vi "test_Create Data Channel_array enumerated list.vi"(8 "error in (no error)":errorcluster, 11 "TestCase in":refnum<class "Instrument Addon Scripting API Channels Unit Tests.lvclass">) -> (0 "error out":errorcluster, 3 "TestCase out":refnum<class "Instrument Addon Scripting API Channels Unit Tests.lvclass">)   [LabVIEW 2020, in "Instrument Addon Scripting API Channels Unit Tests.lvclass"]
uses:
  Instrument Addon Scripting API Channels Unit Tests.lvclass
  APIs/Scripting API/TypeDefs/Array Enumerated List Settings.ctl
  APIs/Scripting API/TypeDefs/Array Element.ctl
  Addon/Addon Shared/Types/Protocol Data Type.ctl
  Addon/Addon Shared/Types/Data Channel Type.ctl
  Instrument Addon Scripting API Channels Unit Tests.lvclass/Instrument Addon Scripting API Channels Unit Tests.ctl
  Addon/Addon Shared/SubVIs/Constants.vi
  <vilib>/NI/NI VeriStand Advanced SysDef API/_SubVIs/SysDef.Search.GUID.vi
  <vilib>/NI/NI VeriStand Advanced SysDef API/_SubVIs/SysDef.Search.GUIDs.vi
  APIs/Scripting API/Channels/Create Data Channel - Array - Enumerated List.vi
  <vilib>/NI VeriStand/Custom Device API/Get Item Property (U16).vi
  <vilib>/addons/_JKI Toolkits/VI Tester/TestCase.llb/TestCase.lvclass
  <vilib>/NI/NI VeriStand Advanced SysDef API/SysDef API/Advanced System Definition.lvlib
  Addon/Addon Shared/Instrument Addon Shared.lvlib
  APIs/Scripting API/Instrument Addon Scripting API.lvlib
  <vilib>/NI VeriStand/Custom Device API/Custom Device API.lvlib
  C:/Program Files (x86)/National Instruments/LabVIEW 2020/vi.lib/addons/_JKI Toolkits/VI Tester/TestCase.llb/TestCase.lvclass
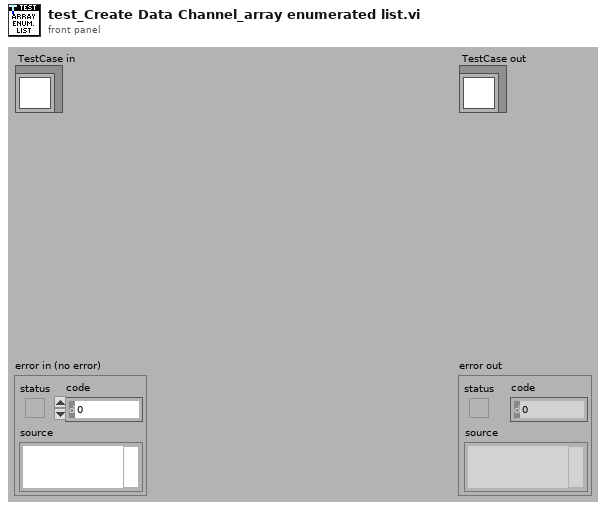
[diagram p1: front panel]
types:
  T1 = typedef "Instrument Addon Scripting API.lvlib/Array Enumerated List Settings.ctl" = cluster{"Elements":T2[], "Enumerated List":string[], "Delimiter":string}
  T2 = typedef "Instrument Addon Scripting API.lvlib/Array Element.ctl" = cluster{"Name":string, "Default Value":dbl, "Units":string}
  T3 = typedef "Instrument Addon Shared.lvlib/Data Channel Type.ctl" = enum16{"Format", "Comparison", "Type Cast", "Enumerated List"}
  T4 = typedef "Instrument Addon Shared.lvlib/Protocol Data Type.ctl" = enum16{"Single Channel", "Array"}
  T5 = typedef "Custom Device API.lvlib/Custom Device Item Ref.ctl" = u64
  T6 = typedef "Advanced System Definition.lvlib/TreeItem.Info.ctl" = cluster{"Name":string, "Description":string, "GUID":string, "Is Channel":bool, "Channel":T7, "Is Waveform":bool, "Waveform":T9}
  T7 = typedef "Custom Device API.lvlib/Custom Device Channel.ctl" = cluster{"Type":T8, "Units":string, "Default Value":dbl, "Faultable":bool, "Scalable":bool}
  T8 = typedef "Custom Device API.lvlib/Custom Device Channel Type.ctl" = enum16{"Input", "Output"}
  T9 = typedef "Custom Device API.lvlib/Custom Device Waveform.ctl" = cluster{"Data Type":T10, "Units":string}
  T10 = typedef "Custom Device API.lvlib/Custom Device Waveform DataType.ctl" = enum16{"Double", "Complex Double"}
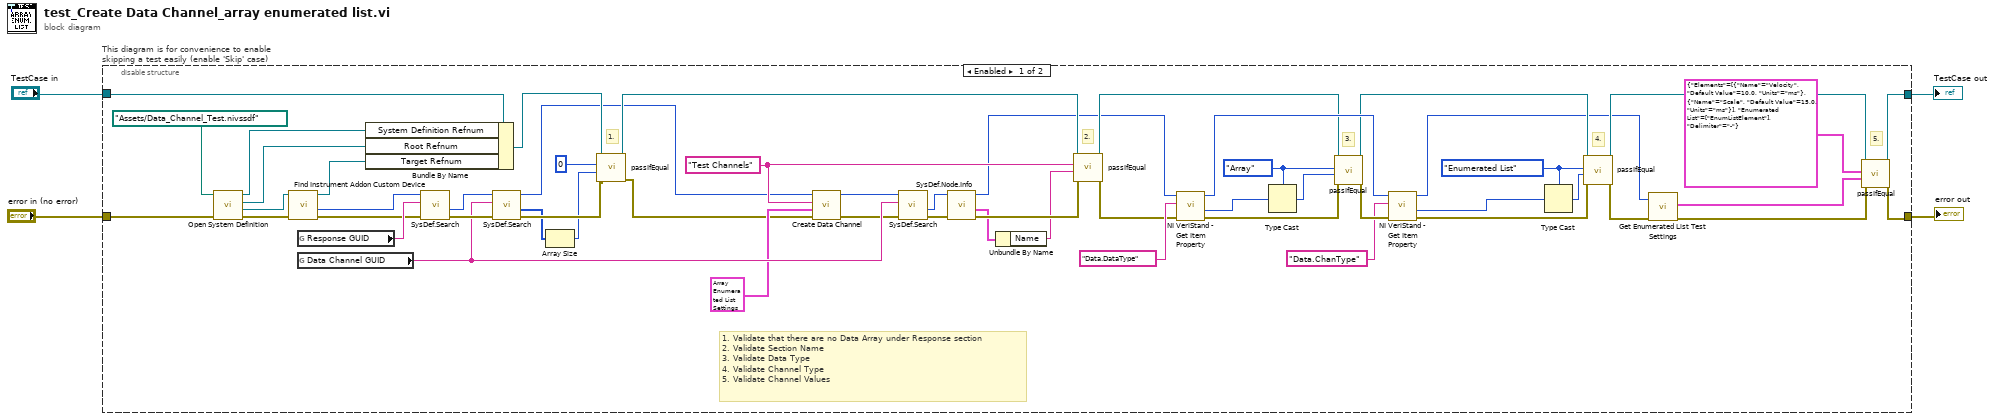
[diagram p0: block diagram]
diagram:
  n1 = disable-structure "This diagram is for convenience to enable skipping a test easily (enable 'Skip' case)" shown="Enabled" {
    disable-tunnel: "TestCase in" -> [w30 w63]
    disable-tunnel: [w36 w61] -> w1
    disable-tunnel: [w37 w62] -> w3
    disable-tunnel: "error in (no error)" -> [w56 w60]
    frame Enabled {
      w16 = Data_Channel_Type."Enumerated List" ("Channel Type")
      w21 = Protocol_Data_Type."Array" ("Data Type")
      w45 = "Test Channels" ("Name")
      # "1. Validate that there are no Data Array under Response section\n2. Validate Section Name\n3. Validate Data Type\n4. Validate Channel Type\n5. Validate Channel Values"
      # "4."
      # "3."
      # "5."
      # "2."
      # "1."
      n2 = call "Open System Definition.vi"("error in (no error)"=w56, "System Definition File"=path "Assets/Data_Channel_Test.nivssdf") -> ("error out"=w59:errorcluster, "Target Refnum"=w58:refnum<k24>, "Root Refnum"=w32:refnum<k24>, "System Definition Refnum"=w33:refnum<k24>)  [unwired: 6 in]
      n3 = call "Find Instrument Addon Custom Device.vi"("error in"=w59, "target in"=w58) -> ("error out"=w28:errorcluster, "NodeID"=w55:u64, "target out"=w31:refnum<k24>)  [unwired: 7 in]
      n4 = global read "Constants.vi" "Response GUID"() -> (w54:string)
      n5 = global read "Constants.vi" "Data Channel GUID"() -> (w51:string)
      n6 = Bundle By Name(cluster=w30, "System Definition Refnum"=w33, "Root Refnum"=w32, "Target Refnum"=w31) -> (w29:refnum<class "Instrument Addon Scripting API Channels Unit Tests.lvclass">)
      n7 = call-poly <vilib>:"SysDef.Search.vi"("error in (no error)"=w28, "GUID"=w54, "nodeID"=w55) -> ("error out"=w52:errorcluster, "Value out"=w53:u64)  [unwired: 5 in, 2 out]
      n8 = call-poly <vilib>:"SysDef.Search.vi"("error in (no error)"=w52, "GUID"=w51, "nodeID"=w53) -> ("error out"=w49:errorcluster, "Values Out"=w48:u64[], "nodeID out"=w5:u64)  [unwired: 5 in, 1 out]
      n9 = Array Size(array=w48) -> (size(s)=w47:i32)
      n10 = call-dynamic "passIfEqual.vi"("error in (no error)"=w49, "y"=w47, "x"=0 ("size(s)"), "TestCase in"=w29) -> ("error out"=w27:errorcluster, "TestCase out"=w50:refnum<class "Instrument Addon Scripting API Channels Unit Tests.lvclass">)  [unwired: 6 in]
      n11 = call-poly "Create Data Channel.vi"("error in (no error)"=w27, "settings"=T1 {"Elements"=[{"Name"="Velocity", "Default Value"=10.0, "Units"="ms"}, {"Name"="Scale", "Default Value"=15.0, "Units"="ms"}], "Enumerated List"=["EnumListElement"], "Delimiter"="-"} ("Settings"), "channel name"=w45, "response refnum in"=w5) -> ("error out"=w44:errorcluster, "response refnum out"=w43:T5)  [unwired: 4 in, 2 out]
      n12 = call-poly <vilib>:"SysDef.Search.vi"("error in (no error)"=w44, "GUID"=w51, "nodeID"=w43) -> ("error out"=w42:errorcluster, "Value out"=w41:u64)  [unwired: 5 in, 2 out]
      n13 = call <vilib>:"SysDef.Node.Info.vi"("error in (no error)"=w42, "nodeID"=w41) -> ("error out"=w40:errorcluster, "Item Info"=w39:T6, "nodeID out"=w8:u64)  [unwired: 6 in, 1 out]
      n14 = Unbundle By Name(w39) -> ("Name"=w38:string)
      n15 = call-dynamic "passIfEqual.vi"("error in (no error)"=w40, "y"=w38, "x"=w45, "TestCase in"=w50) -> ("error out"=w11:errorcluster, "TestCase out"=w13:refnum<class "Instrument Addon Scripting API Channels Unit Tests.lvclass">)  [unwired: 6 in]
      n16 = call-poly <vilib>:"NI VeriStand - Get Item Property.vi"("error in (no error)"=w11, "Property Name"="Data.DataType", "Item Ref in"=w8) -> ("error out"=w24:errorcluster, "Value"=w23:u16, "Item Ref out"=w15:T5)  [unwired: 5 in, 1 out]
      n17 = Type Cast(type=w21, x=w23) -> (*(type *) &x=w22:T4)
      n18 = call-dynamic "passIfEqual.vi"("error in (no error)"=w24, "y"=w22, "x"=w21, "TestCase in"=w13) -> ("error out"=w20:errorcluster, "TestCase out"=w12:refnum<class "Instrument Addon Scripting API Channels Unit Tests.lvclass">)  [unwired: 6 in]
      n19 = call-poly <vilib>:"NI VeriStand - Get Item Property.vi"("error in (no error)"=w20, "Property Name"="Data.ChanType", "Item Ref in"=w15) -> ("error out"=w19:errorcluster, "Value"=w18:u16, "Item Ref out"=w9:T5)  [unwired: 5 in, 1 out]
      n20 = Type Cast(type=w16, x=w18) -> (*(type *) &x=w17:T3)
      n21 = call-dynamic "passIfEqual.vi"("error in (no error)"=w19, "y"=w17, "x"=w16, "TestCase in"=w12) -> ("error out"=w7:errorcluster, "TestCase out"=w10:refnum<class "Instrument Addon Scripting API Channels Unit Tests.lvclass">)  [unwired: 6 in]
      n22 = call "Get Enumerated List Test Settings.vi"("Error In"=w7, "Data Channel Ref In"=w9) -> ("Error Out"=w35:errorcluster, "Data Channel Settings"=w6:T1)  [unwired: 7 in, 1 out]
      n23 = call-dynamic "passIfEqual.vi"("error in (no error)"=w35, "y"=w6, "x"=T1 {"Elements"=[{"Name"="Velocity", "Default Value"=10.0, "Units"="ms"}, {"Name"="Scale", "Default Value"=15.0, "Units"="ms"}], "Enumerated List"=["EnumListElement"], "Delimiter"="-"} ("Settings"), "TestCase in"=w10) -> ("error out"=w37:errorcluster, "TestCase out"=w36:refnum<class "Instrument Addon Scripting API Channels Unit Tests.lvclass">)  [unwired: 6 in]
    }
    frame Disabled {
      # "skip test result while test is under development"
      n24 = call <vilib>:"skip.vi"("error in (no error)"=w60, "TestCase in"=w63) -> ("error out"=w62:errorcluster, "TestCase out"=w61:refnum<class "Instrument Addon Scripting API Channels Unit Tests.lvclass">)  [unwired: 8 in]
    }
  }
  "error out" <- w3
  "TestCase out" <- w1
